vi "STM Write Message (Serial).vi"(6 "Options":T1={"Ignore Timeout Error"=TRUE, "timeout ms (1000)"=1000}, 8 "error in (no error)":errorcluster, 9 "Data":string, 10 "Name":string, 11 "Connection Info":T2) -> (0 "error out":errorcluster, 3 "Connection Info Out":T2)   [LabVIEW 2014, in "QwaveSys Raspberry Pi Library.lvlib"]
doc: "This VI writes a package of data to a remote computer. It prepends a meta data ID number to each packet. \n\nThe data must be passed in as a String. The calling VI is responsible for flattening the desired data to a string before passing it to this VI."
uses:
  QwaveSys Raspberry Pi Library.lvlib
  stm_Serial Connection Info.ctl
  _SubVIs/stm_MetaDataElement.ctl
  stm_Serial Write Options.ctl
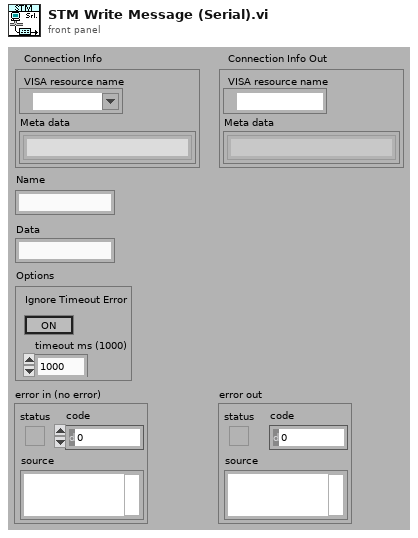
[diagram p1: front panel]
types:
  T1 = typedef "QwaveSys Raspberry Pi Library.lvlib/stm_Serial Write Options.ctl" = cluster{"Ignore Timeout Error":bool, "timeout ms (1000)":u32}
  T2 = typedef "QwaveSys Raspberry Pi Library.lvlib/stm_Serial Connection Info.ctl" = cluster{"VISA resource name":refnum<visa-resource-name>, "Meta data":T3[]}
  T3 = typedef "QwaveSys Raspberry Pi Library.lvlib/stm_MetaDataElement.ctl" = string
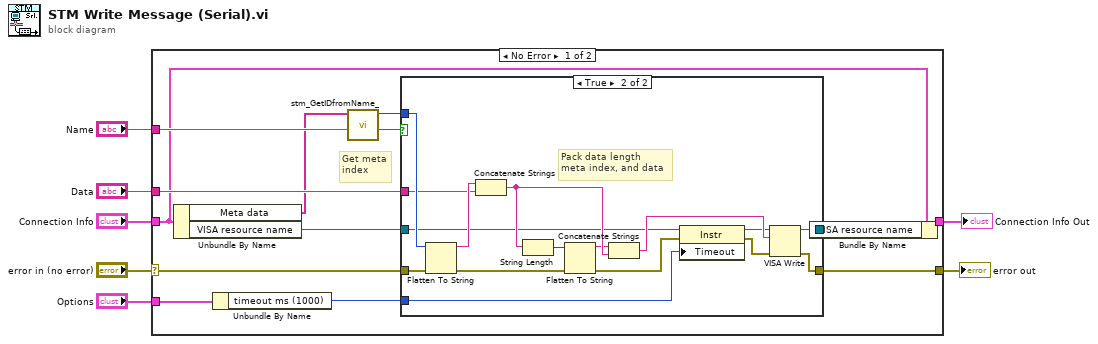
[diagram p0: block diagram]
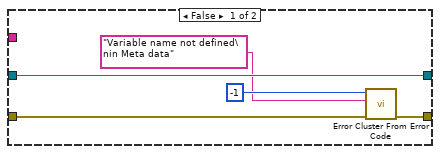
[diagram p2: hidden frame]
diagram:
  n1 = case shown="No Error" "error in (no error)" {
    selector: "error in (no error)" -> [w15 w43]
    tunnel: "Connection Info" -> [w10 w42]
    tunnel: [w20 w43] -> w6
    tunnel: [w9 w42] -> w5
    tunnel: "Name" -> [w19 _]
    tunnel: "Data" -> [w17 _]
    tunnel: "Options" -> [w14 _]
    frame No Error {
      # "Get meta\nindex"
      n2 = Unbundle By Name(w10) -> ("Meta data"=w11:T3[], "VISA resource name"=w12:refnum<visa-resource-name>)
      n3 = Unbundle By Name(w14) -> ("timeout ms (1000)"=w13:u32)
      n4 = call "stm_GetIDfromName_.vi"("Name"=w19, "MetaData"=w11) -> ("Found"=w16:bool, "Meta ID"=w18:u16)  [unwired: 8 out]
      n5 = case shown="True" w16 {
        tunnel: w12 -> [w25 w30]
        tunnel: w15 -> [w24 w32]
        tunnel: [w23 w41] -> w20
        tunnel: [w25 w40] -> w8
        tunnel: w18 -> [_ w39]
        tunnel: w17 -> [_ w35]
        tunnel: w13 -> [_ w28]
        frame False {
          n6 = call <vilib>:"Error Cluster From Error Code.vi"("error in (no error)"=w24, "error message (\"\")"="Variable name not defined\nin Meta data" ("source"), "error code (0)"=-1) -> ("error out"=w23:errorcluster)  [unwired: 1 in, 5 out]
        }
        frame True {
          # "Pack data length\nmeta index, and data"
          n7 = Flatten To String(anything=w39, error in (no error)=w32) -> (data string=w38:string, error out=w31:errorcluster)  [unwired: 3 out]
          n8 = Concatenate Strings(w38, w35) -> (w36:string)
          n9 = String Length(string=w36) -> (length=w37:i32)
          n10 = Flatten To String(anything=w37, error in (no error)=w31) -> (data string=w34:string, error out=w29:errorcluster)  [unwired: 3 out]
          n11 = Concatenate Strings(w34, w36) -> (w33:string)
          n12 = property class="Instr"(reference=w30, error in=w29, "Timeout"=w28) -> (reference out=w26:refnum<visa-resource-name>, error out=w27:errorcluster)
          n13 = VISA Write(VISA resource name=w26, write buffer=w33, error in (no error)=w27) -> (VISA resource name out=w40:refnum<visa-resource-name>, error out=w41:errorcluster)  [unwired: 1 out]
        }
      }
      n14 = Bundle By Name(cluster=w10, "VISA resource name"=w8) -> (w9:T2)
    }
    frame Error {
    }
  }
  "error out" <- w6
  "Connection Info Out" <- w5
